vi "CSC_ExtForce2Torque.vi"(5 "BodyWtComp?(F)":bool, 7 "CuffWtComp?(F)":bool=TRUE, 8 "error in (no error)":errorcluster, 9 "ExternalForce(T)":bool=TRUE, 10 "External Force (In GCS)":T1, 11 "CSC in":refnum<class "CableSerialChain.lvclass">) -> (0 "error out":errorcluster, 2 "DesiredTorque(Nm)":dbl[](array[numeric]), 3 "CSC out":refnum<class "CableSerialChain.lvclass">)   [LabVIEW 2015, in "CableSerialChain.lvclass"]
uses:
  CableSerialChain.lvclass
  Body/Force.ctl
  Body/PointOnBody.ctl
  CableSerialChain.lvclass/CableSerialChain.ctl
  <vilib>/Analysis/BLAS.llb/dgemv - General Matrix-Vector Product (DBL).vi
  <vilib>/Utility/error.llb/Error Cluster From Error Code.vi
  Body/Bodies.lvclass
  <vilib>/Analysis/NI_AALBLAS.lvlib
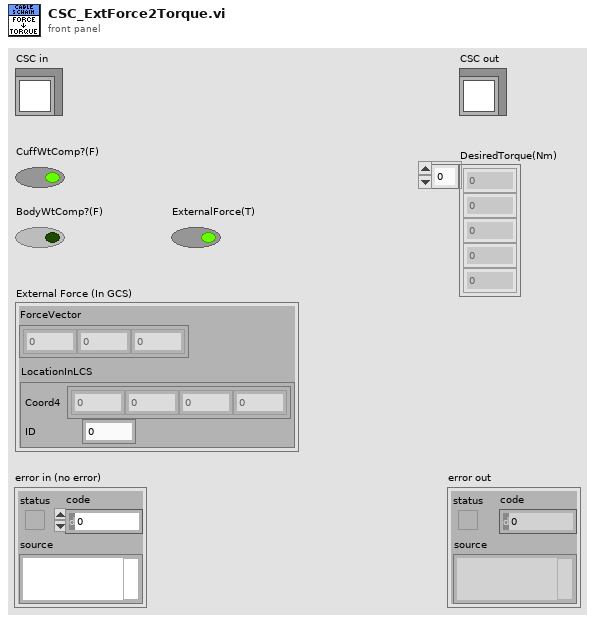
[diagram p1: front panel]
types:
  T1 = typedef "Bodies.lvclass/Force.ctl" = cluster{"LocationInLCS":T2, "ForceVector":dbl[]}
  T2 = typedef "Bodies.lvclass/PointOnBody.ctl" = cluster{"Coord4":dbl[], "ID":i32}
  T3 = typedef "CableSerialChain.lvclass/Cuff.ctl" = cluster{"BodyID":i32, "CoM(CuffCS)":T2, "Mass(kg)":dbl, "CablePts(CuffCS)":T2[], "Cuff->Body":T4}
  T4 = typedef "NI_Matrix.lvlib/RealMatrix.ctl" = dbl[][]
  T5 = cluster{cluster{"dgemv":dbl[], "BodyID":i32}, "GravityVector":dbl[]}
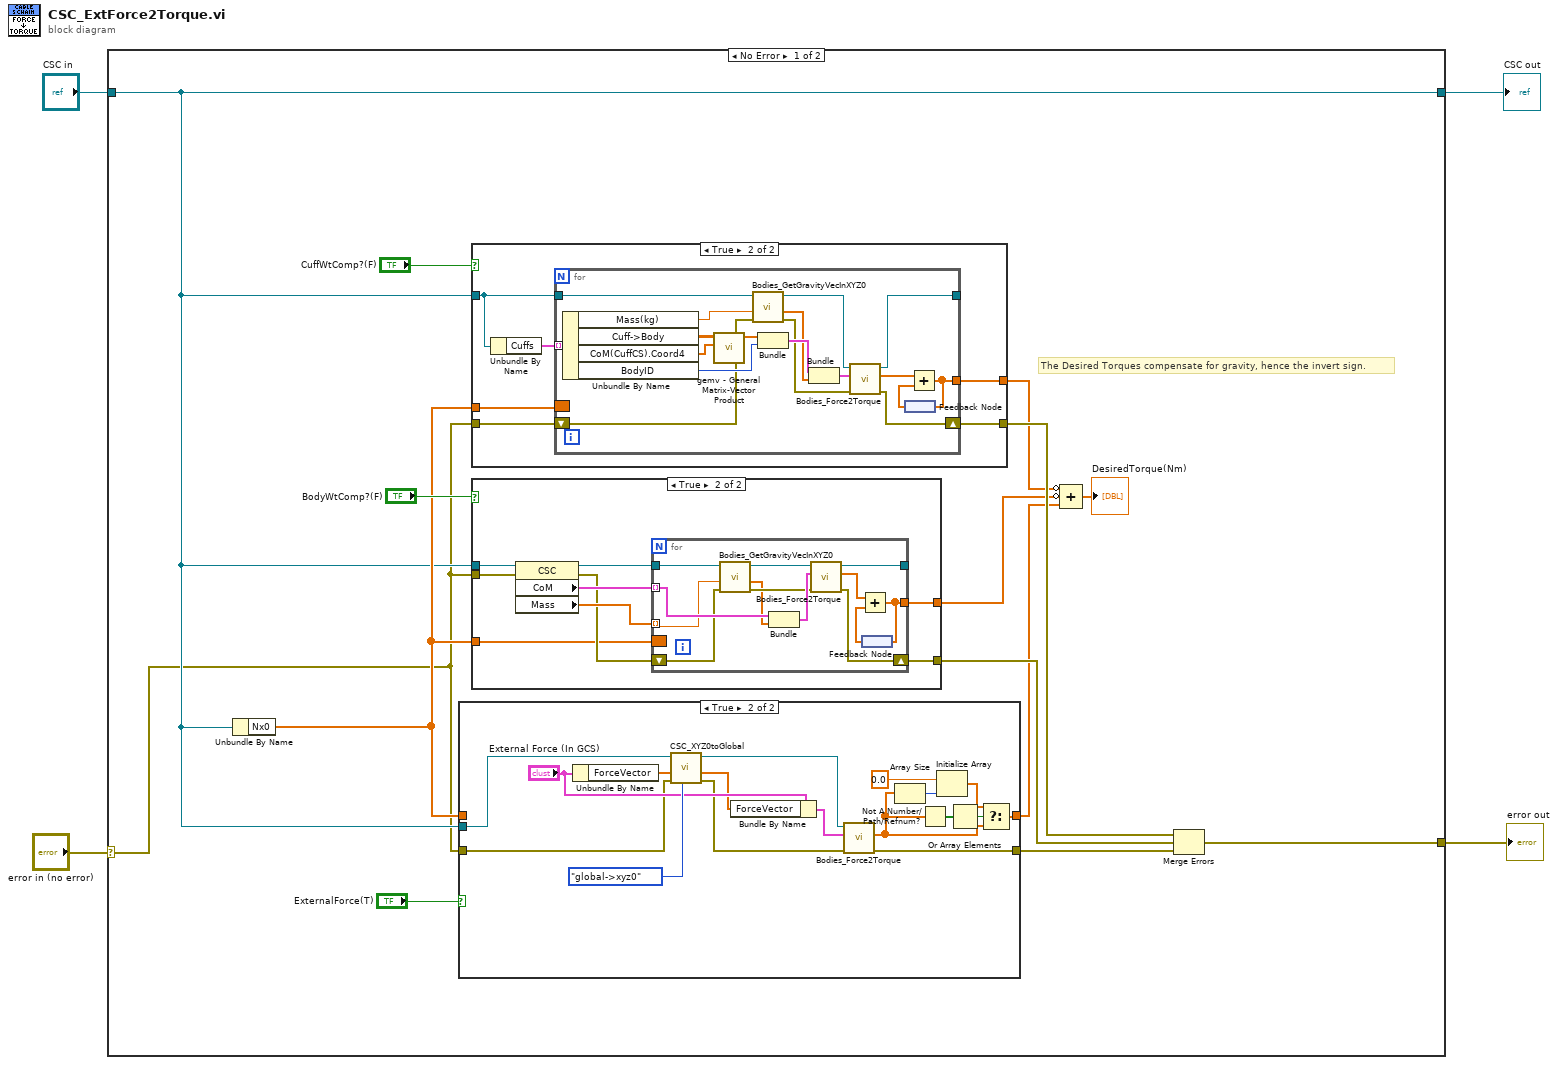
[diagram p0: block diagram]
diagram:
  n1 = case shown="No Error" "error in (no error)" {
    selector: "error in (no error)" -> [w5 w89]
    tunnel: [w14 w89] -> w3
    tunnel: [w6 w88] -> w1
    tunnel: "CSC in" -> [w6 w88]
    frame No Error {
      # "The Desired Torques compensate for gravity, hence the invert sign."
      n2 = Unbundle By Name(w6) -> ("Nx0"=w7:dbl[])
      n3 = case shown="True" "ExternalForce(T)" {
        tunnel: [w19 w37] -> w17
        tunnel: w6 -> [_ w24]
        tunnel: w5 -> [w19 w22]
        tunnel: [w20 w36] -> w9
        tunnel: w7 -> [w20 _]
        frame False {
        }
        frame True {
          n4 = Unbundle By Name("External Force (In GCS)") -> ("ForceVector"=w28:dbl[])
          n5 = call "CSC_XYZ0toGlobal.vi"("Dir(xyz0->global)"=enum16{"global->xyz0", "xyz0->global"}."global->xyz0", "error in (no error)"=w22, "Vin"=w28, "CSC In"=w24) -> ("error out"=w21:errorcluster, "Vout"=w26:dbl[], "CSC Oout"=w23:refnum<class "CableSerialChain.lvclass">)  [unwired: 4 in, 1 out]
          n6 = Bundle By Name(cluster="External Force (In GCS)", "ForceVector"=w26) -> (w25:T1)
          n7 = call "Bodies_Force2Torque.vi"("error in (no error)"=w21, "Force"=w25, "Bodies.lvclass"=w23) -> ("error out"=w37:errorcluster, "Torque Vector"=w32:dbl[])  [unwired: 5 in, 2 out]
          n8 = Array Size(array=w32) -> (size(s)=w33:i32)
          n9 = Not A Number/Path/Refnum?(number/path/refnum=w32) -> (NaN/Path/Refnum?=w35:bool[])
          n10 = Initialize Array(0.0 ("element"), w33) -> (w30:dbl[])
          n11 = Or Array Elements(Boolean array=w35) -> (logical OR=w34:bool)
          n12 = Select(t=w30, s=w34, f=w32) -> (s? t:f=w36:dbl[])
        }
      }
      n13 = case shown="True" "CuffWtComp?(F)" {
        tunnel: w6 -> [_ w64]
        tunnel: w5 -> [w62 w69]
        tunnel: [w62 w68] -> w15
        tunnel: [w63 w67] -> w13
        tunnel: w7 -> [w63 w66]
        frame False {
        }
        frame True {
          n14 = Unbundle By Name(w64) -> ("Cuffs"=w65:T3[])
          n15 = for {
            tunnel: w65 -> [w87] mode=indexing
            tunnel: [w83] -> w67
            border: w66 -> [_]
            shift-right: [w82] -> w68
            shift-left: w69 -> [w70]
            tunnel: w64 -> [w75]
            tunnel: [w86] -> _
            n16 = Unbundle By Name(w87) -> ("Mass(kg)"=w73:dbl, "Cuff->Body"=w81:T4, "CoM(CuffCS).Coord4"=w80:dbl[], "BodyID"=w77:i32)
            n17 = call-poly <vilib>:"gemv - General Matrix-Vector Product.vi"("x"=w80, "A"=w81) -> ("dgemv"=w78:dbl[])  [unwired: 8 in, 1 out]
            n18 = call "Bodies_GetGravityVecInXYZ0.vi"("error in (no error)"=w70, "Mass(kg)"=w73, "Bodies in"=w75) -> ("error out"=w71:errorcluster, "GravityVector"=w72:dbl[], "Bodies out"=w74:refnum<class "CableSerialChain.lvclass">)  [unwired: 6 in]
            n19 = Bundle("dgemv"=w78, "BodyID"=w77) -> (w76:cluster{"dgemv":dbl[], "BodyID":i32})  [unwired: 1 in]
            n20 = Bundle(w76, "GravityVector"=w72) -> (w79:T5)  [unwired: 1 in]
            n21 = call "Bodies_Force2Torque.vi"("error in (no error)"=w71, "Force"=w79, "Bodies.lvclass"=w74) -> ("error out"=w82:errorcluster, "Torque Vector"=w85:dbl[], "Bodies.lvclass 2"=w86:refnum<class "CableSerialChain.lvclass">)  [unwired: 5 in, 1 out]
            n22 = feedback #1() -> (w84:dbl[])
            n23 = Add(x=w85, y=w84) -> (x+y=w83:dbl[])
            n24 = feedback-in #1(w83) -> ()
          }
        }
      }
      n25 = case shown="True" "BodyWtComp?(F)" {
        tunnel: [w38 w44] -> w16
        tunnel: w6 -> [_ w43]
        tunnel: w5 -> [w38 w42]
        tunnel: [w39 w41] -> w11
        tunnel: w7 -> [w39 w40]
        frame False {
        }
        frame True {
          n26 = property class="CSC"(reference=w43, error in=w42) -> (reference out=w46:refnum<class "CableSerialChain.lvclass">, error out=w45:errorcluster, "CoM"=w48:T2[], "Mass"=w47:dbl[])
          n27 = for {
            tunnel: w48 -> [w60] mode=indexing
            tunnel: w47 -> [w50] mode=indexing
            shift-right: [w58] -> w44
            shift-left: w45 -> [w54]
            border: w40 -> [_]
            tunnel: [w56] -> w41
            tunnel: w46 -> [w52]
            tunnel: [w61] -> _
            n28 = call "Bodies_GetGravityVecInXYZ0.vi"("error in (no error)"=w54, "Mass(kg)"=w50, "Bodies in"=w52) -> ("error out"=w53:errorcluster, "GravityVector"=w49:dbl[], "Bodies out"=w51:refnum<class "CableSerialChain.lvclass">)  [unwired: 6 in]
            n29 = Bundle("Point"=w60, "GravityVector"=w49) -> (w59:cluster{"Point":T2, "GravityVector":dbl[]})  [unwired: 1 in]
            n30 = call "Bodies_Force2Torque.vi"("error in (no error)"=w53, "Force"=w59, "Bodies.lvclass"=w51) -> ("error out"=w58:errorcluster, "Torque Vector"=w55:dbl[], "Bodies.lvclass 2"=w61:refnum<class "CableSerialChain.lvclass">)  [unwired: 5 in, 1 out]
            n31 = feedback #2() -> (w57:dbl[])
            n32 = Add(x=w55, y=w57) -> (x+y=w56:dbl[])
            n33 = feedback-in #2(w56) -> ()
          }
        }
      }
      n34 = Compound Arithmetic op=ADD(invert w13, invert w11, w9) -> (→"DesiredTorque(Nm)":dbl[])
      n35 = Merge Errors(w15, w16, w17) -> (w14:errorcluster)
    }
    frame Error {
    }
  }
  "error out" <- w3
  "CSC out" <- w1
